vi "WS1050_Extract Data From Scope_T1_T2_T3.vi"(0 "file path":path=path "S:/_Employee_Folders/Andy temp/SN01/444AB_04__SN01_C1_S1_UP_Switch_Time_data.csv", 1 "60% Amp":dbl=0.6, 2 "95% Amp":dbl=0.95, 9 "Set Point for AMP":i32=7000, 11 "error in (no error)":errorcluster, 12 "90% Amp":dbl=0.9) -> (3 "AMP(v)":dbl=1.1, 4 "Amp(mv)":string, 6 "T2(us)":string, 8 "T3(us)":string, 10 "T1(us)":string, 13 "Signal":dbl[](graph), 14 "Filtered Signal":dbl[](graph), 15 "error out":errorcluster)   [LabVIEW 2017]
uses:
  <vilib>/Utility/file.llb/Read From Spreadsheet File (string).vi
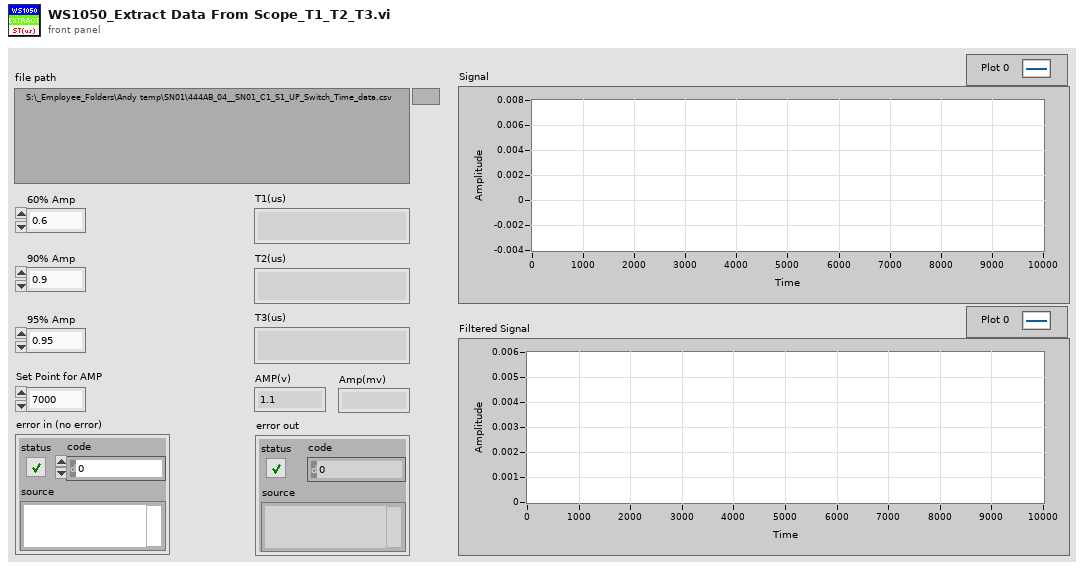
[diagram p1: front panel]
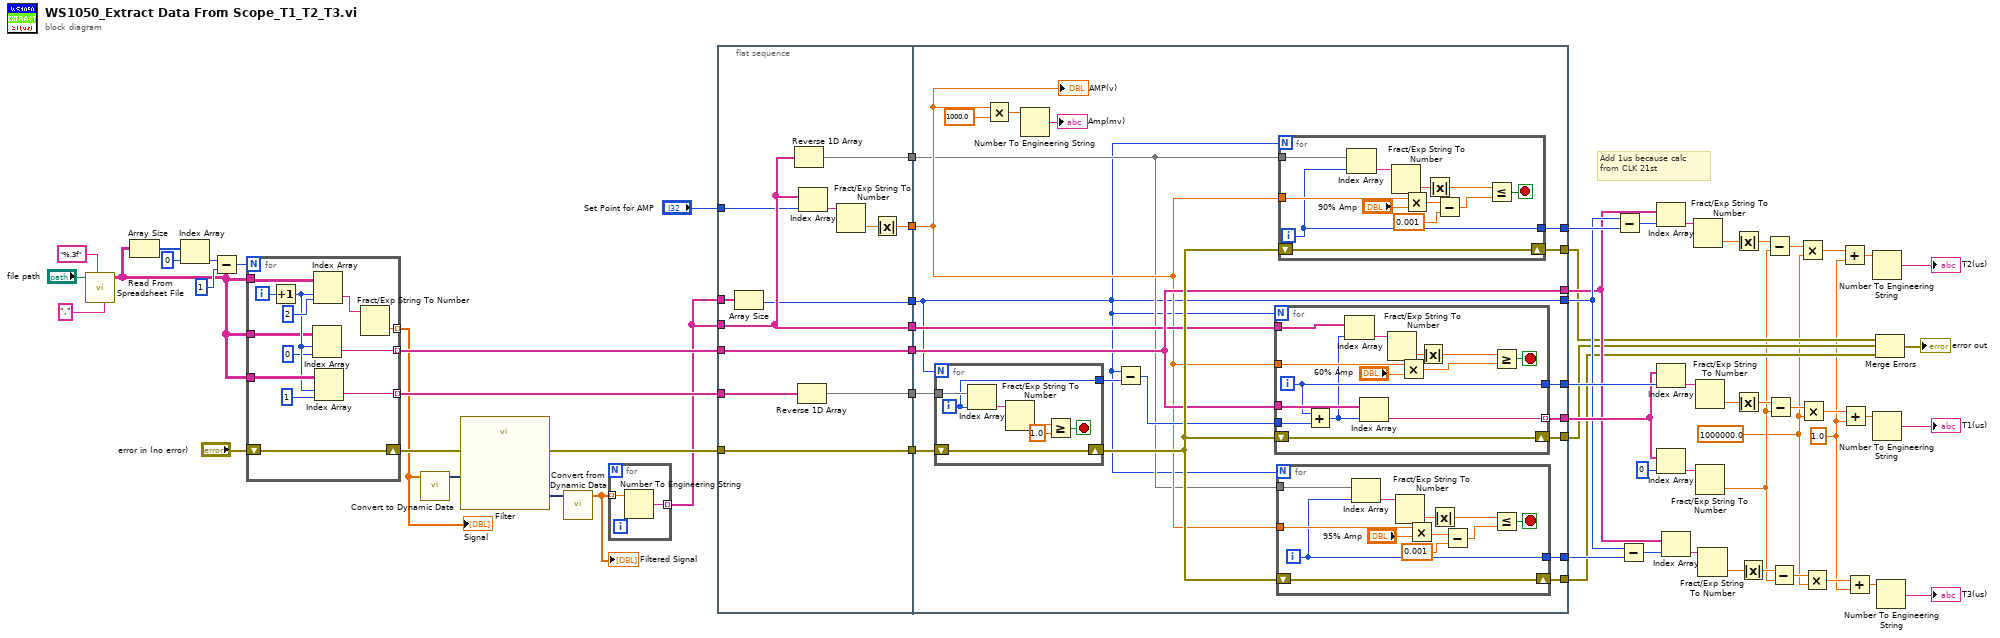
[diagram p0: block diagram]
diagram:
  w1 = 1.0 ("y")
  w2 = 1000000.0 ("y")
  # "Add 1us because calc \nfrom CLK 21st"
  n1 = call-poly <vilib>:"Read From Spreadsheet File.vi"("delimiter (\\t)"="," ("delimiter (\\t)"), "format (%s)"="%.3f" ("format (%.3f)"), "file path (dialog if empty)"="file path") -> ("all rows"=w49:string[][])  [unwired: 4 in, 4 out]
  n2 = Array Size(array=w49) -> (size(s)=w62:i32[])
  n3 = Index Array(array=w62, index=0) -> (element=w60:i32)
  n4 = Subtract(x=w60, y=1) -> (x-y=w50:i32)
  n5 = for {
    N: w50 -> [_]
    tunnel: w49 -> [w78]
    tunnel: w49 -> [w75]
    tunnel: [w73] -> w57 mode=indexing
    tunnel: w49 -> [w71]
    tunnel: [w69] -> w51 mode=indexing
    shift-right: [w68] -> w33
    shift-left: "error in (no error)" -> [w68]
    tunnel: [w66] -> w28 mode=indexing
    i -> [w76]
    n6 = Increment(x=w76) -> (x+1=w72:i32)
    n7 = Index Array(array=w71, index (row)=w72, index (col)=0 ("disabled index (col)")) -> (element=w69:string)
    n8 = Index Array(array=w78, index (row)=w72, index (col)=2 ("disabled index (col)")) -> (element=w67:string)
    n9 = Index Array(array=w75, index (row)=w72, index (col)=1 ("disabled index (col)")) -> (element=w73:string)
    n10 = Fract/Exp String To Number(string=w67) -> (number=w66:dbl)  [unwired: 3 in, 1 out]
  }
  "Signal" <- w28
  n11 = call "Convert to Dynamic Data"("Array"=w28) -> ("Dynamic Data Type"=w32:dynamicdata)  [unwired: 3 in]
  n12 = call "Filter"("error in (no error)"=w33, "Signal"=w32) -> ("error out"=w31:errorcluster, "Filtered Signal"=w30:dynamicdata)  [unwired: 8 in]
  n13 = call "Convert from Dynamic Data"("Dynamic Data Type"=w30) -> ("Array"=w26:dbl[])  [unwired: 3 in]
  "Filtered Signal" <- w26
  n14 = for {
    tunnel: w26 -> [w80] mode=indexing
    tunnel: [w79] -> w29 mode=indexing
    n15 = Number To Engineering String(4:w80) -> (0:w79:string)  [unwired: 3 in]
  }
  n16 = flat-sequence {
    tunnel: w51 -> [w91]
    tunnel: w31 -> [w92]
    tunnel: w57 -> [w87]
    tunnel: [w92] -> w40
    tunnel: [w91] -> w39
    tunnel: w29 -> [w84]
    tunnel: [w88] -> w38
    tunnel: [w86] -> w37
    tunnel: [w85] -> w36
    tunnel: [w84] -> w35
    tunnel: [w83] -> w34
    tunnel: w29 -> [w82]
    tunnel: "Set Point for AMP" -> [w81]
    tunnel: [w112] -> w58
    tunnel: [w110] -> w44
    tunnel: [w109] -> w43
    tunnel: [w105] -> w53
    tunnel: [w104] -> w52
    tunnel: [w93] -> w46
    tunnel: [w99] -> w45
    tunnel: [w101] -> w42
    tunnel: [w100] -> w47
    tunnel: w40 -> [w111]
    tunnel: w39 -> [w99]
    tunnel: w38 -> [w96]
    tunnel: w37 -> [w95]
    tunnel: w36 -> [w94]
    tunnel: w35 -> [w97]
    tunnel: w34 -> [w93]
    frame #0 {
      n17 = Array Size(array=w82) -> (size(s)=w83:i32)
      n18 = Reverse 1D Array(array=w84) -> (reversed array=w85:string[])
      n19 = Reverse 1D Array(array=w87) -> (reversed array=w86:string[])
      n20 = Index Array(array=w84, index=w81) -> (element=w89:string)
      n21 = Fract/Exp String To Number(string=w89) -> (number=w90:dbl)  [unwired: 3 in, 1 out]
      n22 = Absolute Value(x=w90) -> (abs(x)=w88:dbl)
    }
    frame #1 {
      n23 = for {
        N: w93 -> [_]
        tunnel: w95 -> [w157]
        tunnel: [w154] -> w103
        shift-right: [w152] -> w102
        shift-left: w111 -> [w152]
        i -> [w154]
        stop <- w155 stop-if-true
        n24 = Index Array(array=w157, index=w154) -> (element=w151:string)
        n25 = Fract/Exp String To Number(string=w151) -> (number=w153:dbl)  [unwired: 3 in, 1 out]
        n26 = Greater Or Equal?(x=w153, y=1.0) -> (x >= y?=w155:bool)
      }
      n27 = Multiply(x=w96, y=1000.0) -> (x*y=w107:dbl)
      n28 = Number To Engineering String(4:w107) -> (0:→"Amp(mv)":string)  [unwired: 3 in]
      n29 = Subtract(x=w93, y=w103) -> (x-y=w98:i32)
      n30 = for {
        N: w93 -> [_]
        tunnel: w97 -> [w150]
        tunnel: w96 -> [w148]
        tunnel: w99 -> [w147]
        tunnel: [w146] -> w104 mode=indexing
        tunnel: [w143] -> w112
        tunnel: w98 -> [w145]
        shift-right: [w140] -> w109
        shift-left: w102 -> [w140]
        i -> [w143]
        stop <- w149 stop-if-true
        n31 = Add(x=w143, y=w145) -> (x+y=w142:i32)
        n32 = Index Array(array=w150, index=w142) -> (element=w144:string)
        n33 = Index Array(array=w147, index=w142) -> (element=w146:string)
        n34 = Fract/Exp String To Number(string=w144) -> (number=w139:dbl)  [unwired: 3 in, 1 out]
        n35 = Multiply(x=w148, y="60% Amp") -> (x*y=w137:dbl)
        n36 = Absolute Value(x=w139) -> (abs(x)=w138:dbl)
        n37 = Greater Or Equal?(x=w138, y=w137) -> (x >= y?=w149:bool)
      }
      n38 = for {
        N: w93 -> [_]
        tunnel: w94 -> [w124]
        tunnel: w96 -> [w122]
        tunnel: [w118] -> w100
        shift-right: [w120] -> w101
        shift-left: w102 -> [w120]
        i -> [w118]
        stop <- w123 stop-if-true
        n39 = Index Array(array=w124, index=w118) -> (element=w117:string)
        n40 = Fract/Exp String To Number(string=w117) -> (number=w119:dbl)  [unwired: 3 in, 1 out]
        n41 = Multiply(x=w122, y="95% Amp") -> (x*y=w115:dbl)
        n42 = Absolute Value(x=w119) -> (abs(x)=w116:dbl)
        n43 = Subtract(x=w115, y=0.001) -> (x-y=w114:dbl)
        n44 = Less Or Equal?(x=w116, y=w114) -> (x <= y?=w123:bool)
      }
      n45 = for {
        N: w93 -> [_]
        tunnel: w94 -> [w136]
        tunnel: w96 -> [w134]
        tunnel: [w130] -> w105
        shift-right: [w132] -> w110
        shift-left: w102 -> [w132]
        i -> [w130]
        stop <- w135 stop-if-true
        n46 = Index Array(array=w136, index=w130) -> (element=w129:string)
        n47 = Fract/Exp String To Number(string=w129) -> (number=w131:dbl)  [unwired: 3 in, 1 out]
        n48 = Multiply(x=w134, y="90% Amp") -> (x*y=w127:dbl)
        n49 = Absolute Value(x=w131) -> (abs(x)=w128:dbl)
        n50 = Subtract(x=w127, y=0.001) -> (x-y=w126:dbl)
        n51 = Less Or Equal?(x=w128, y=w126) -> (x <= y?=w135:bool)
      }
      "AMP(v)" <- w96
    }
  }
  n52 = Subtract(x=w46, y=w53) -> (x-y=w11:i32)
  n53 = Subtract(x=w46, y=w47) -> (x-y=w10:i32)
  n54 = Index Array(array=w45, index=w11) -> (element=w20:string)
  n55 = Index Array(array=w52, index=w58) -> (element=w25:string)
  n56 = Index Array(array=w52, index=0) -> (element=w23:string)
  n57 = Index Array(array=w45, index=w10) -> (element=w5:string)
  n58 = Fract/Exp String To Number(string=w20) -> (number=w14:dbl)  [unwired: 3 in, 1 out]
  n59 = Fract/Exp String To Number(string=w25) -> (number=w12:dbl)  [unwired: 3 in, 1 out]
  n60 = Fract/Exp String To Number(string=w23) -> (number=w3:dbl)  [unwired: 3 in, 1 out]
  n61 = Fract/Exp String To Number(string=w5) -> (number=w9:dbl)  [unwired: 3 in, 1 out]
  n62 = Absolute Value(x=w14) -> (abs(x)=w15:dbl)
  n63 = Absolute Value(x=w12) -> (abs(x)=w13:dbl)
  n64 = Absolute Value(x=w9) -> (abs(x)=w8:dbl)
  n65 = Subtract(x=w15, y=w3) -> (x-y=w21:dbl)
  n66 = Subtract(x=w13, y=w3) -> (x-y=w22:dbl)
  n67 = Subtract(x=w8, y=w3) -> (x-y=w4:dbl)
  n68 = Multiply(x=w21, y=w2) -> (x*y=w16:dbl)
  n69 = Multiply(x=w22, y=w2) -> (x*y=w18:dbl)
  n70 = Multiply(x=w4, y=w2) -> (x*y=w7:dbl)
  n71 = Add(x=w16, y=w1) -> (x+y=w17:dbl)
  n72 = Add(x=w18, y=w1) -> (x+y=w19:dbl)
  n73 = Add(x=w7, y=w1) -> (x+y=w6:dbl)
  n74 = Number To Engineering String(4:w17) -> (0:→"T2(us)":string)  [unwired: 3 in]
  n75 = Number To Engineering String(4:w19) -> (0:→"T1(us)":string)  [unwired: 3 in]
  n76 = Merge Errors(w44, w43, w42) -> (→"error out":errorcluster)
  n77 = Number To Engineering String(4:w6) -> (0:→"T3(us)":string)  [unwired: 3 in]
